vi "getFileNAme.vi"(11 "Path":path) -> (2 "filenames":string[](array[string]), 3 "appended path":path)   [LabVIEW 2013]
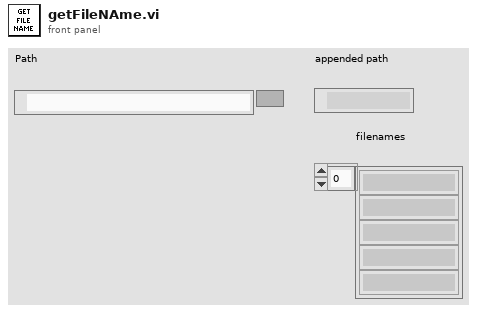
[diagram p1: front panel]
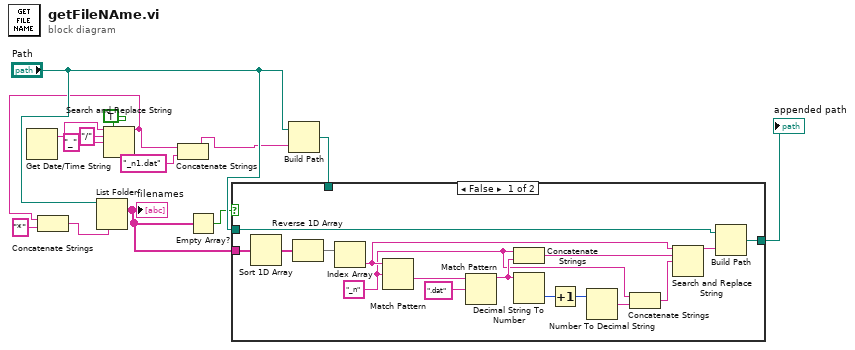
[diagram p0: block diagram]
diagram:
  n1 = Get Date/Time String() -> (date string=w1:string)  [unwired: 3 in, 1 out]
  n2 = Search and Replace String(replace all?=TRUE ("replace all? (F)"), input string=w1, search string="/", replace string="_" ("replace string (\"\")")) -> (result string=w9:string)  [unwired: 4 in, 3 out]
  n3 = Concatenate Strings(w9, "*" ("string")) -> (w7:string)
  n4 = List Folder(path="Path", pattern=w7) -> (filenames=w8:string[])  [unwired: 2 in, 3 out]
  "filenames" <- w8
  n5 = Concatenate Strings(w9, "_n1.dat" ("string")) -> (w5:string)
  n6 = Empty Array?(array=w8) -> (empty?=w11:bool)
  n7 = Build Path(base path="Path", name or relative path=w5) -> (appended path=w12:path)
  n8 = case shown="False" w11 {
    tunnel: w8 -> [w30 _]
    tunnel: "Path" -> [w18 _]
    tunnel: [w17 w31] -> w14
    tunnel: w12 -> [_ w31]
    frame False {
      w22 = "_n"
      n9 = Sort 1D Array(array=w30) -> (sorted array=w16:string[])
      n10 = Reverse 1D Array(array=w16) -> (reversed array=w15:string[])
      n11 = Index Array(array=w15) -> (element=w24:string)  [unwired: 1 in]
      n12 = Match Pattern(string=w24, regular expression=w22) -> (after substring=w28:string)  [unwired: 1 in, 3 out]
      n13 = Match Pattern(string=w28, regular expression=".dat") -> (before substring=w25:string)  [unwired: 1 in, 3 out]
      n14 = Concatenate Strings(w22, w25) -> (w23:string)
      n15 = Decimal String To Number(string=w25) -> (number=w27:i32)  [unwired: 2 in, 1 out]
      n16 = Increment(x=w27) -> (x+1=w26:i32)
      n17 = Number To Decimal String(number=w26) -> (decimal integer string=w21:string)  [unwired: 1 in]
      n18 = Concatenate Strings(w22, w21) -> (w20:string)
      n19 = Search and Replace String(input string=w24, search string=w23, replace string=w20) -> (result string=w19:string)  [unwired: 5 in, 3 out]
      n20 = Build Path(base path=w18, name or relative path=w19) -> (appended path=w17:path)
    }
    frame True {
    }
  }
  "appended path" <- w14
